vi "Write Ctl Refnum.vi"(4 "Error In":errorcluster, 6 "Ctl Refnum":refnum<vi>, 7 "Font Settting in":refnum<class "Display Properties.lvclass">) -> (0 "Error Out":errorcluster, 3 "Font Settting out":refnum<class "Display Properties.lvclass">)   [LabVIEW 2015, in "Display Properties Manager.lvlib" / "Display Properties.lvclass"]
uses:
  Display Properties.lvclass
  Display Properties.lvclass/Display Properties.ctl
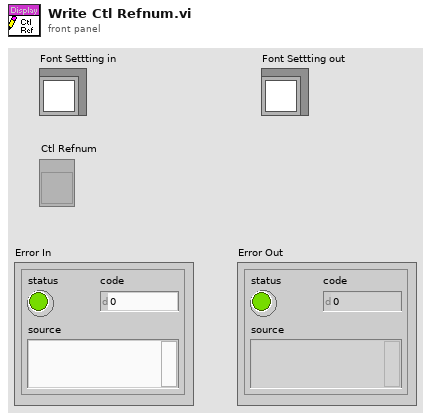
[diagram p1: front panel]
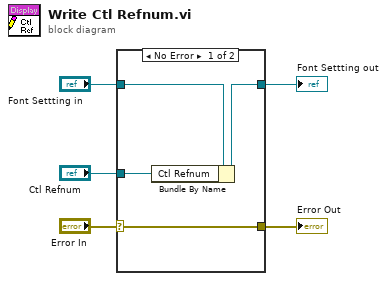
[diagram p0: block diagram]
diagram:
  n1 = case shown="No Error" "Error In" {
    selector: "Error In" -> [w9 w10]
    tunnel: [w9 w10] -> w4
    tunnel: [w7 w11] -> w2
    tunnel: "Font Settting in" -> [w8 w11]
    tunnel: "Ctl Refnum" -> [w6 _]
    frame No Error {
      n2 = Bundle By Name(cluster=w8, "Ctl Refnum"=w6) -> (w7:refnum<class "Display Properties.lvclass">)
    }
    frame Error {
    }
  }
  "Error Out" <- w4
  "Font Settting out" <- w2
